vi "Init Active Devices.vi"(8 "error in":errorcluster, 10 "Device Names":string, 11 "DAC Keller Diff P 23X in":refnum<class "DAC Keller Diff P 23X.lvclass">) -> (0 "error out":errorcluster, 3 "DAC Keller Diff P 23X out":refnum<class "DAC Keller Diff P 23X.lvclass">)   [LabVIEW 2019, in "DAC.lvlib" / "DAC Keller Diff P 23X.lvclass"]
uses:
  DAC Keller Diff P 23X.lvclass
  C:/Users/wg/Documents/LV_Projects/test-stand/App/DAC/DAC.lvclass
  DAC.lvclass/DAC.ctl
  DAC Keller Diff P 23X.lvclass/DAC Keller Diff P 23X.ctl
  DAC.lvclass
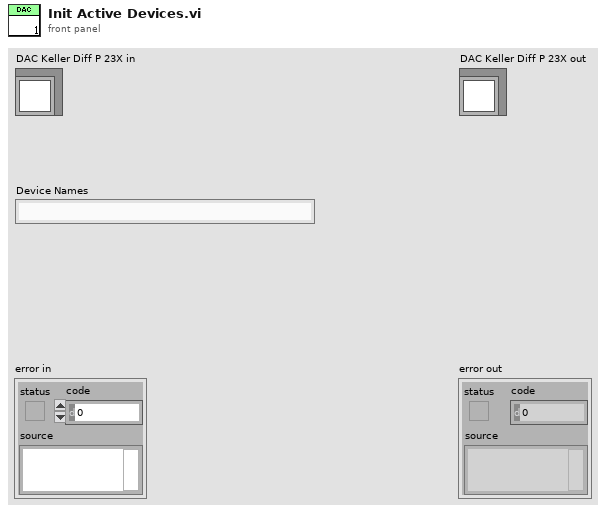
[diagram p1: front panel]
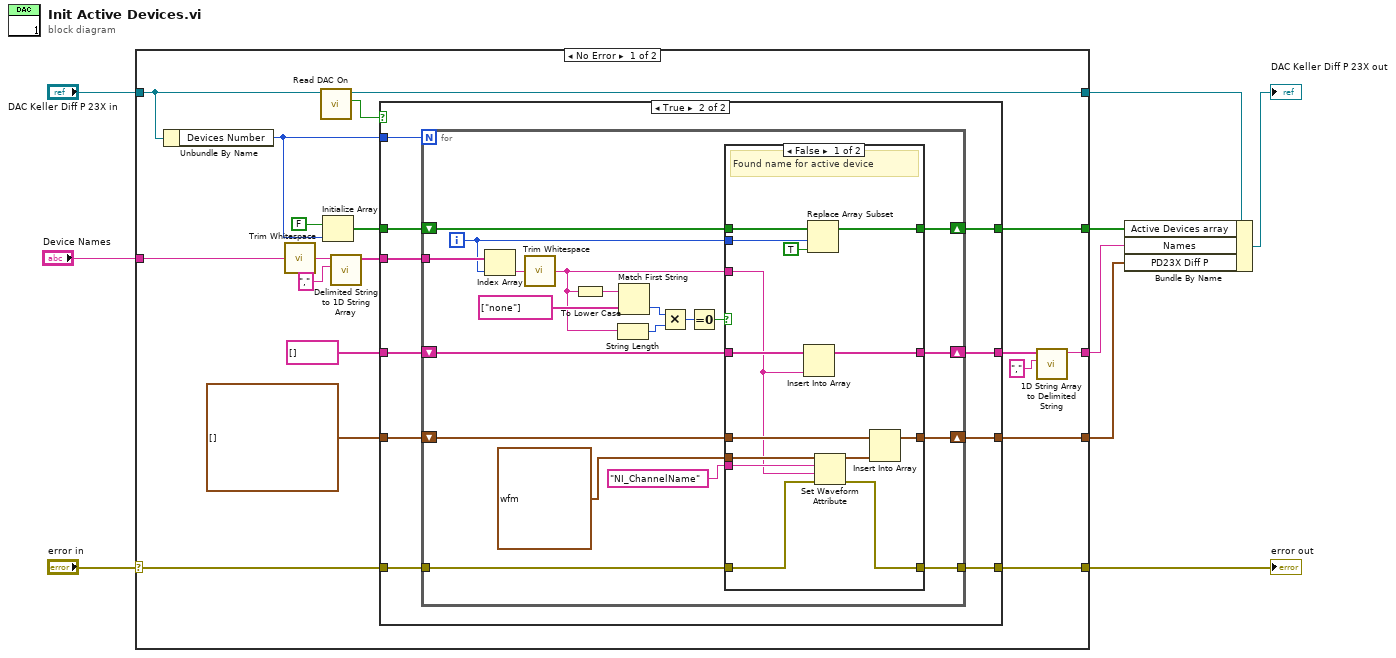
[diagram p0: block diagram]
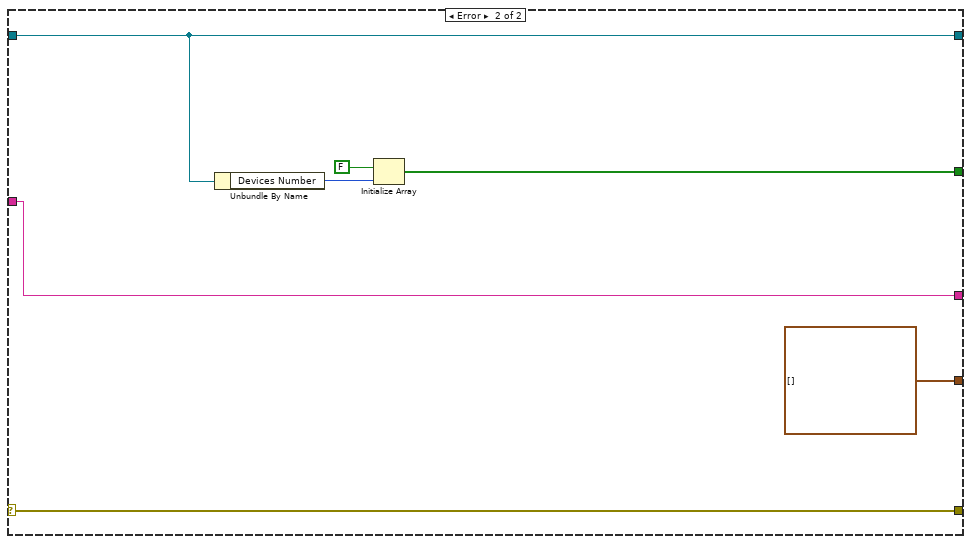
[diagram p4: hidden frame]
diagram:
  n1 = case shown="No Error" "error in" {
    selector: "error in" -> [w12 w87]
    tunnel: [w11 w87] -> w8
    tunnel: [w20 w84] -> w6
    tunnel: "DAC Keller Diff P 23X in" -> [w21 w84]
    tunnel: [w22 w83] -> w3
    tunnel: "Device Names" -> [w18 w82]
    tunnel: [w14 w82] -> w2
    tunnel: [w10 waveform(sgl)[] []] -> w1
    frame No Error {
      n2 = Unbundle By Name(w21) -> ("Devices Number"=w24:i32)
      n3 = call <vilib>:"Trim Whitespace.vi"("string"=w18) -> ("trimmed string"=w28:string)  [unwired: 1 in]
      n4 = call "Read DAC On.vi"("DAC in"=w21) -> ("DAC On"=w19:bool, "DAC out"=w20:refnum<class "DAC Keller Diff P 23X.lvclass">)  [unwired: 8 in, 1 out]
      n5 = Initialize Array(FALSE, w24) -> (w23:bool[])
      n6 = call <vilib>:"Delimited String to 1D String Array.vi"("delimiter"=",", "delimited string"=w28) -> ("string array"=w25:string[])  [unwired: 9 in]
      n7 = case shown="True" w19 {
        tunnel: w25 -> [w31 w42]
        tunnel: w24 -> [_ w41]
        tunnel: w23 -> [w32 w40]
        tunnel: [w32 w39] -> w22
        tunnel: string[] [] -> [_ w38]
        tunnel: [w31 w37] -> w16
        tunnel: waveform(sgl)[] [] -> [w30 w36]
        tunnel: [w30 w35] -> w10
        tunnel: w12 -> [w29 w34]
        tunnel: [w29 w33] -> w11
        frame False {
        }
        frame True {
          n8 = for {
            N: w41 -> [_]
            tunnel: w42 -> [w62]
            shift-right: [w53] -> w39
            shift-left: w40 -> [w54]
            shift-right: [w51] -> w37
            shift-left: w38 -> [w52]
            shift-right: [w47] -> w35
            shift-left: w36 -> [w48]
            tunnel: w34 -> [w44]
            tunnel: [w43] -> w33
            i -> [w55]
            n9 = Index Array(array=w62, index=w55) -> (element=w61:string)
            n10 = call <vilib>:"Trim Whitespace.vi"("string"=w61) -> ("trimmed string"=w49:string)  [unwired: 1 in]
            n11 = To Lower Case(string=w49) -> (all lower case string=w50:string)
            n12 = String Length(string=w49) -> (length=w59:i32)
            n13 = Match First String(2:string[] ["none"], 3:w50) -> (0:w58:i32)  [unwired: 1 out]
            n14 = Multiply(x=w58, y=w59) -> (x*y=w57:i32)
            n15 = Equal To 0?(x=w57) -> (x = 0?=w56:bool)
            n16 = case shown="False" w56 {
              tunnel: w49 -> [w65 _]
              tunnel: w55 -> [w75 _]
              tunnel: w54 -> [w76 w80]
              tunnel: [w73 w80] -> w53
              tunnel: w52 -> [w72 w79]
              tunnel: [w71 w79] -> w51
              tunnel: w48 -> [w70 w78]
              tunnel: [w69 w78] -> w47
              tunnel: waveform(sgl) {"t0"=timestamp(0 s since 1904-01-01), "dt"=1.0, "Y"=[]} ("Waveform") -> [w67 _]
              tunnel: "NI_ChannelName" ("name") -> [w66 _]
              tunnel: w44 -> [w64 w77]
              tunnel: [w63 w77] -> w43
              frame False {
                # "Found name for active device"
                n17 = Insert Into Array "Insert Into Array"(array=w72, new element=w65) -> (w71:string[])  [unwired: 1 in]
                n18 = Replace Array Subset "Replace Array Subset"(array=w76, new element=TRUE ("new element/subarray"), index=w75) -> (w73:bool[])
                n19 = Set Waveform Attribute(4:w64, 5:w65, 6:w66, 7:w67) -> (0:w63:errorcluster, 3:w68:waveform(sgl))  [unwired: 1 out]
                n20 = Insert Into Array "Insert Into Array"(array=w70, new element=w68) -> (w69:waveform(sgl)[])  [unwired: 1 in]
              }
              frame True {
                # "Empty or 'none' - inactive device"
              }
            }
          }
        }
      }
      n21 = call <vilib>:"1D String Array to Delimited String.vi"("delimiter"=",", "string array"=w16) -> ("delimited string"=w14:string)  [unwired: 9 in]
    }
    frame Error {
      n22 = Unbundle By Name(w84) -> ("Devices Number"=w85:i32)
      n23 = Initialize Array(FALSE, w85) -> (w83:bool[])
    }
  }
  "error out" <- w8
  n24 = Bundle By Name(cluster=w6, "Active Devices array"=w3, "Names"=w2, "PD23X Diff P"=w1) -> (→"DAC Keller Diff P 23X out":refnum<class "DAC Keller Diff P 23X.lvclass">)
